vi "Example Callback.vi"() -> ()   [LabVIEW 2010]
uses:
  C:/tf/play/labview/Tinkerforge.dll
  Tinkerforge.dll
panel:
  in  "stop":bool
  in  "uid":string="63oL6P"
  in  "port":i32=4223
  in  "host":string="localhost"
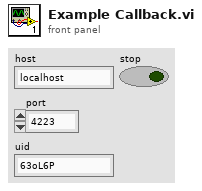
[diagram p1: front panel]
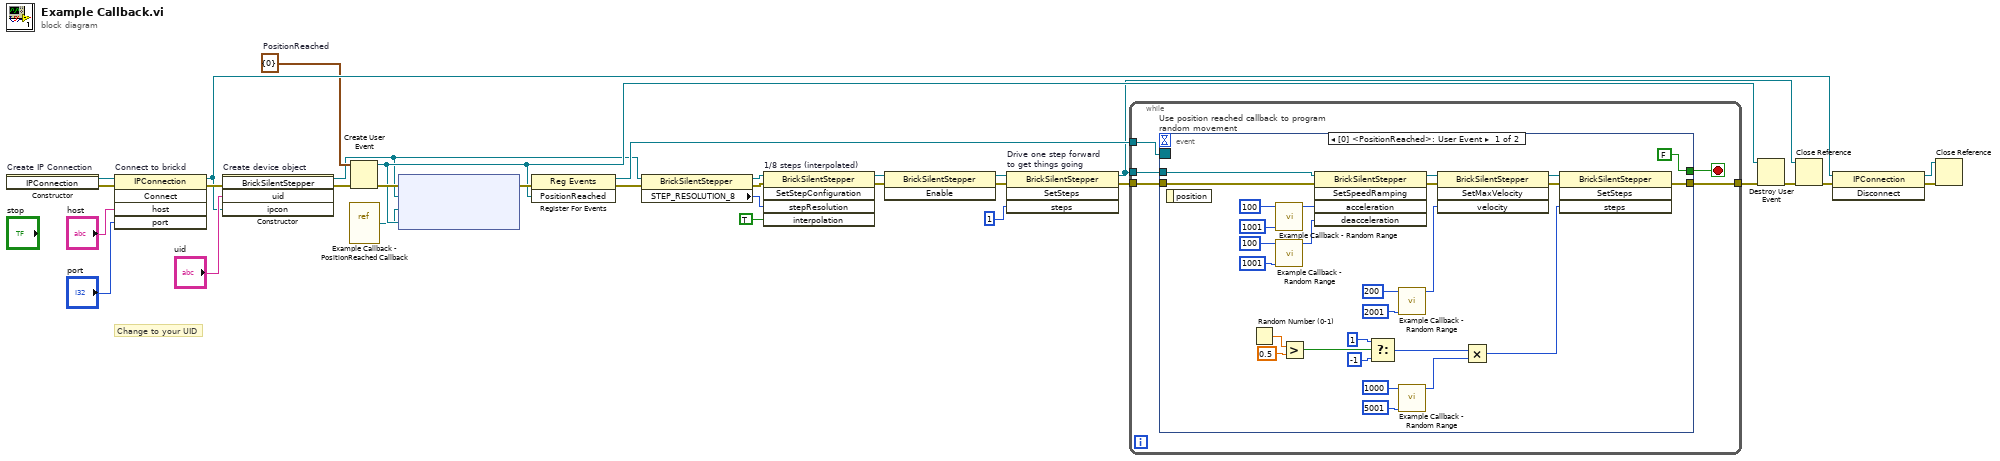
[diagram p0: block diagram]
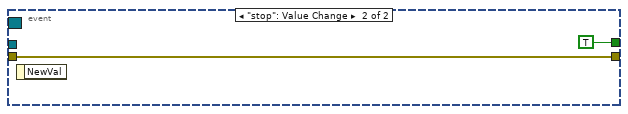
[diagram p2: hidden frame]
diagram:
  w17 = cluster{"position":i32} {"position"=0}  # PositionReached
  # "Change to your UID"
  n1 = constructor on="Create IP Connection" class="IPConnection"() -> (reference out=w32:refnum<k24>, error out=w10:errorcluster)  [unwired: 3 in, 1 out]
  n2 = invoke on="Connect to brickd" class="IPConnection" method="Connect"(reference=w32, error in=w10, "host"="host", "port"="port") -> (reference out=w25:refnum<k24>, error out=w28:errorcluster)  [unwired: 1 in, 3 out]
  n3 = constructor on="Create device object" class="BrickSilentStepper"(error in=w28, "uid"="uid", "ipcon"=w25) -> (reference out=w6:refnum<k24>, error out=w16:errorcluster)  [unwired: 2 in, 3 out]
  n4 = vi-ref "Example Callback - PositionReached Callback.vi"() -> ("vi reference"=w9:refnum<vi>)
  n5 = Create User Event(user event datatype=w17, error in=w16) -> (user event=w19:refnum<user-event>, error out=w23:errorcluster)
  n6 = node ("Register Event Callback")(w23, w6, w9, w19) -> (w22:errorcluster)  [unwired: 1 in, 1 out]
  n7 = register-events(error in=w22, w19) -> (reference out=w21:refnum<event-registration>, error out=w3:errorcluster)  [unwired: 1 in]
  n8 = property class="BrickSilentStepper"(reference=w6, error in=w3) -> (reference out=w5:refnum<k24>, error out=w4:errorcluster, "STEP_RESOLUTION_8"=w2:u8)
  n9 = invoke on="1/8 steps (interpolated)" class="BrickSilentStepper" method="SetStepConfiguration"(reference=w5, error in=w4, "stepResolution"=w2, "interpolation"=TRUE) -> (reference out=w7:refnum<k24>, error out=w8:errorcluster)  [unwired: 1 in, 3 out]
  n10 = invoke class="BrickSilentStepper" method="Enable"(reference=w7, error in=w8) -> (reference out=w15:refnum<k24>, error out=w14:errorcluster)  [unwired: 1 in, 1 out]
  n11 = invoke on="Drive one step forward\nto get things going" class="BrickSilentStepper" method="SetSteps"(reference=w15, error in=w14, "steps"=1) -> (reference out=w11:refnum<k24>, error out=w13:errorcluster)  [unwired: 1 in, 2 out]
  n12 = while {
    tunnel: w21 -> [w37]
    tunnel: [w36] -> w20
    tunnel: w13 -> [w35]
    tunnel: w11 -> [w34]
    stop <- w33 stop-if-true
    n13 = event "Use position reached callback to program random movement" shown="[0] <PositionReached>: User Event" {
      selector: w37 -> [_ _]
      dyn-events: _ -> [_ _]
      timeout: _ -> [_ _]
      tunnel: [w64 w65] -> w36
      tunnel: w35 -> [w60 w65]
      tunnel: w34 -> [w39 _]
      tunnel: [FALSE TRUE] -> w33
      event User Event {
        n14 = event-data() -> ()  [unwired: 1 in, 1 out]
        n15 = Random Number (0-1)() -> (number: 0 to 1=w47:dbl)
        n16 = call "Example Callback - Random Range.vi"("max"=1001, "min"=100) -> ("random"=w58:i32)  [unwired: 9 in]
        n17 = call "Example Callback - Random Range.vi"("max"=1001, "min"=100) -> ("random"=w57:i32)  [unwired: 9 in]
        n18 = Greater?(x=w47, y=0.5) -> (0:w45:bool)
        n19 = invoke class="BrickSilentStepper" method="SetSpeedRamping"(reference=w39, error in=w60, "acceleration"=w58, "deacceleration"=w57) -> (reference out=w61:refnum<k24>, error out=w59:errorcluster)  [unwired: 1 in, 3 out]
        n20 = Select(t=1, s=w45, f=-1) -> (s? t:f=w42:i32)
        n21 = call "Example Callback - Random Range.vi"("max"=2001, "min"=200) -> ("random"=w52:i32)  [unwired: 9 in]
        n22 = call "Example Callback - Random Range.vi"("max"=5001, "min"=1000) -> ("random"=w41:i32)  [unwired: 9 in]
        n23 = invoke class="BrickSilentStepper" method="SetMaxVelocity"(reference=w61, error in=w59, "velocity"=w52) -> (reference out=w63:refnum<k24>, error out=w62:errorcluster)  [unwired: 1 in, 2 out]
        n24 = Multiply(x=w42, y=w41) -> (x*y=w40:i32)
        n25 = invoke class="BrickSilentStepper" method="SetSteps"(reference=w63, error in=w62, "steps"=w40) -> (error out=w64:errorcluster)  [unwired: 1 in, 3 out]
      }
      event "stop": Value Change {
        n26 = event-data() -> ()  [unwired: 1 in, 1 out]
      }
    }
  }
  n27 = Destroy User Event(user event=w19, error in=w20) -> (error out=w18:errorcluster)
  n28 = Close Reference(reference=w11, error in (no error)=w18) -> (error out=w27:errorcluster)
  n29 = invoke class="IPConnection" method="Disconnect"(reference=w25, error in=w27) -> (reference out=w24:refnum<k24>, error out=w26:errorcluster)  [unwired: 1 in, 1 out]
  n30 = Close Reference(reference=w24, error in (no error)=w26) -> ()  [unwired: 1 out]
